vi "100 SubVIs 1.vi"() -> ()   [LabVIEW 2018]
panel:
  in  "stop":bool
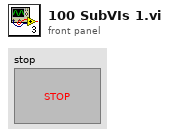
[diagram p1: front panel]
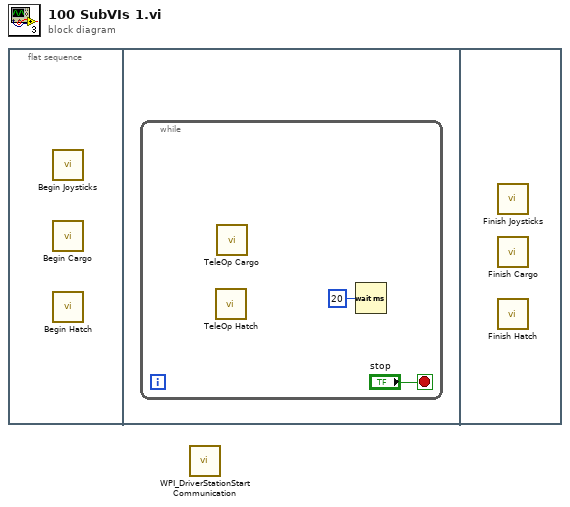
[diagram p0: block diagram]
diagram:
  n1 = flat-sequence {
    frame #0 {
      n2 = call "Begin Joysticks.vi"() -> ()  [unwired: 12 in]
      n3 = call "Begin Cargo.vi"() -> ()  [unwired: 12 in]
      n4 = call "Begin Hatch.vi"() -> ()  [unwired: 12 in]
    }
    frame #1 {
      n5 = while {
        stop <- "stop" stop-if-true
        n6 = call "TeleOp Hatch.vi"() -> ()  [unwired: 12 in]
        n7 = call "TeleOp Cargo.vi"() -> ()  [unwired: 12 in]
        n8 = Wait (ms)(milliseconds to wait=u32 20) -> ()  [unwired: 1 out]
      }
    }
    frame #2 {
      n9 = call "Finish Joysticks.vi"() -> ()  [unwired: 12 in]
      n10 = call "Finish Cargo.vi"() -> ()  [unwired: 12 in]
      n11 = call "Finish Hatch.vi"() -> ()  [unwired: 12 in]
    }
  }
  n12 = call <vilib>:"WPI_DriverStationStart Communication.vi"() -> ()  [unwired: 12 in]
